vi "MCCPMTrestart.vi"(0 "MCCPMT in":refnum<class "MCCPMT.lvclass">, 5 "milliseconds to wait":u32=1000, 11 "error in (no error)":errorcluster) -> (4 "MCCPMT out":refnum<class "MCCPMT.lvclass">, 6 "PMT1 V":dbl, 8 "PMT2 V":dbl, 10 "PMT3 V":dbl, 15 "error out":errorcluster)   [LabVIEW 2012, in "MCCPMT.lvclass"]
uses:
  MCCPMT.lvclass
  MCCPMT.lvclass/MCCPMT.ctl
  <vilib>/ULx/Create Channel.llb/ULx Create Channel (AO-Voltage-Basic).vi
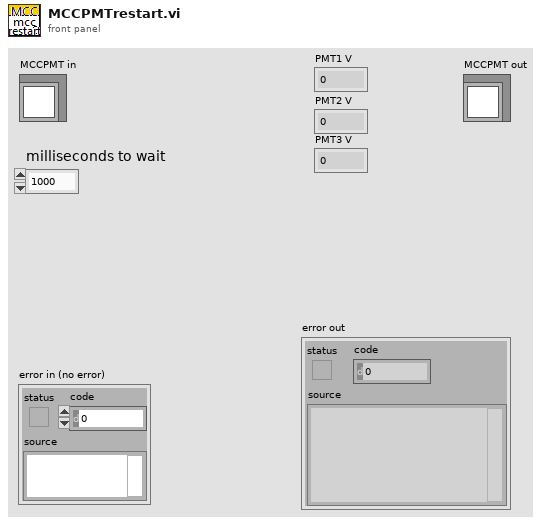
[diagram p1: front panel]
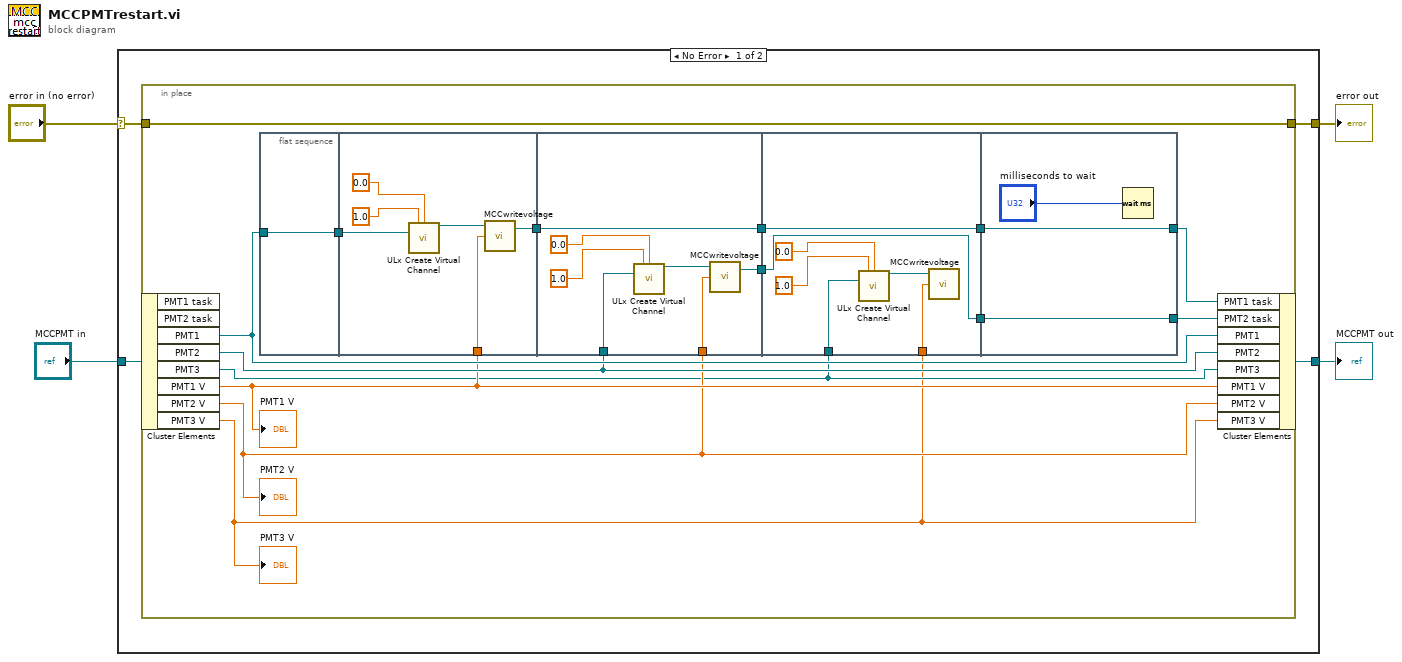
[diagram p0: block diagram]
diagram:
  n1 = case shown="No Error" "error in (no error)" {
    selector: "error in (no error)" -> [w6 w49]
    tunnel: [w5 w49] -> w3
    tunnel: [w7 w48] -> w1
    tunnel: "MCCPMT in" -> [w8 w48]
    frame No Error {
      n2 = in-place {
        in-place-border: w6 -> [w23]
        in-place-border: [w23] -> w5
        n3 = in-place-cluster #1(w8) -> ("PMT1"=w22:refnum<k21>, "PMT2"=w20:refnum<k21>, "PMT3"=w10:refnum<k21>, "PMT1 V"=w16:dbl, "PMT2 V"=w15:dbl, "PMT3 V"=w9:dbl)  [unwired: 2 out]
        "PMT1 V" <- w16
        "PMT2 V" <- w15
        "PMT3 V" <- w9
        n4 = flat-sequence {
          tunnel: w22 -> [w24]
          tunnel: [w24] -> w17
          tunnel: [w26] -> w21
          tunnel: w17 -> [w29]
          tunnel: w16 -> [w25]
          tunnel: w21 -> [w37]
          tunnel: w20 -> [w34]
          tunnel: w15 -> [w31]
          tunnel: [w37] -> w14
          tunnel: [w32] -> w12
          tunnel: w14 -> [w44]
          tunnel: [w44] -> w13
          tunnel: w12 -> [w43]
          tunnel: [w43] -> w11
          tunnel: w10 -> [w39]
          tunnel: w9 -> [w38]
          tunnel: [w46] -> w18
          tunnel: [w47] -> w19
          tunnel: w13 -> [w47]
          tunnel: w11 -> [w46]
          frame #0 {
          }
          frame #1 {
            n5 = call-poly <vilib>:"ULx Create Virtual Channel.vi"("maximum value"=1.0, "minimum value"=0.0, "physical channels"=w29) -> ("task out"=w30:refnum<k24>)  [unwired: 11 in, 1 out]
            n6 = call "MCCwritevoltage.vi"("output voltage"=w25, "task in"=w30) -> ("task out"=w26:refnum<k24>)  [unwired: 1 in, 1 out]
          }
          frame #2 {
            n7 = call-poly <vilib>:"ULx Create Virtual Channel.vi"("maximum value"=1.0, "minimum value"=0.0, "physical channels"=w34) -> ("task out"=w33:refnum<k24>)  [unwired: 11 in, 1 out]
            n8 = call "MCCwritevoltage.vi"("output voltage"=w31, "task in"=w33) -> ("task out"=w32:refnum<k24>)  [unwired: 1 in, 1 out]
          }
          frame #3 {
            n9 = call-poly <vilib>:"ULx Create Virtual Channel.vi"("maximum value"=1.0, "minimum value"=0.0, "physical channels"=w39) -> ("task out"=w40:refnum<k24>)  [unwired: 11 in, 1 out]
            n10 = call "MCCwritevoltage.vi"("output voltage"=w38, "task in"=w40) -> ()  [unwired: 1 in, 2 out]
          }
          frame #4 {
            n11 = Wait (ms)(milliseconds to wait="milliseconds to wait") -> ()  [unwired: 1 out]
          }
        }
        n12 = in-place-cluster #1("PMT1 task"=w19, "PMT2 task"=w18, "PMT1"=w22, "PMT2"=w20, "PMT3"=w10, "PMT1 V"=w16, "PMT2 V"=w15, "PMT3 V"=w9) -> (w7:refnum<class "MCCPMT.lvclass">)
      }
    }
    frame Error {
    }
  }
  "error out" <- w3
  "MCCPMT out" <- w1
